vi "Write.Data.vi"(8 "error in (no error)":errorcluster, 10 "Data":u64[](array[numeric]), 11 "FpgaRunner in":refnum<class "FpgaRunner.lvclass">) -> (0 "error out":errorcluster, 3 "FpgaRunner out":refnum<class "FpgaRunner.lvclass">)   [LabVIEW 2020, in "FpgaRunner.lvclass"]
uses:
  FpgaRunner.lvclass
  FpgaRunner.lvclass/FpgaRunner.ctl
  <vilib>/Utility/error.llb/Error Cluster From Error Code.vi
  <vilib>/rvi/errors/niLvFpgaAdjustHostInterfaceError.vi
  <vilib>/rvi/interface/nirviMethod/nirviMethod.xnode
  <vilib>/FPGAPlugInAG/Dynamic/niLvFpga_WriteFifo_Dynamic.vi
  <vilib>/rvi/errors/niLvFpgaMergeErrorWithErrorCode.vi
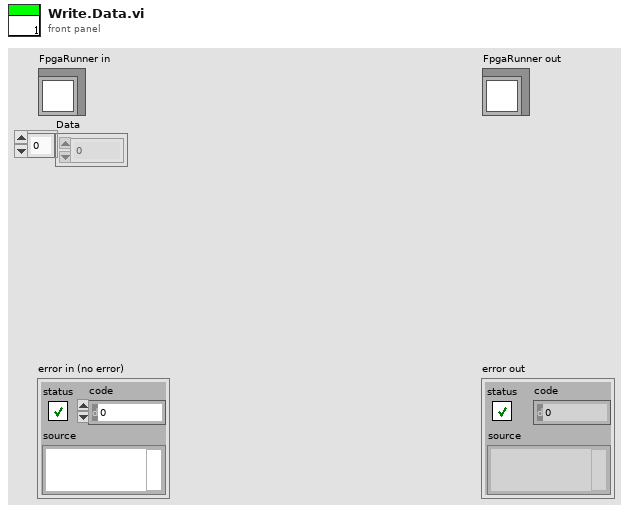
[diagram p1: front panel]
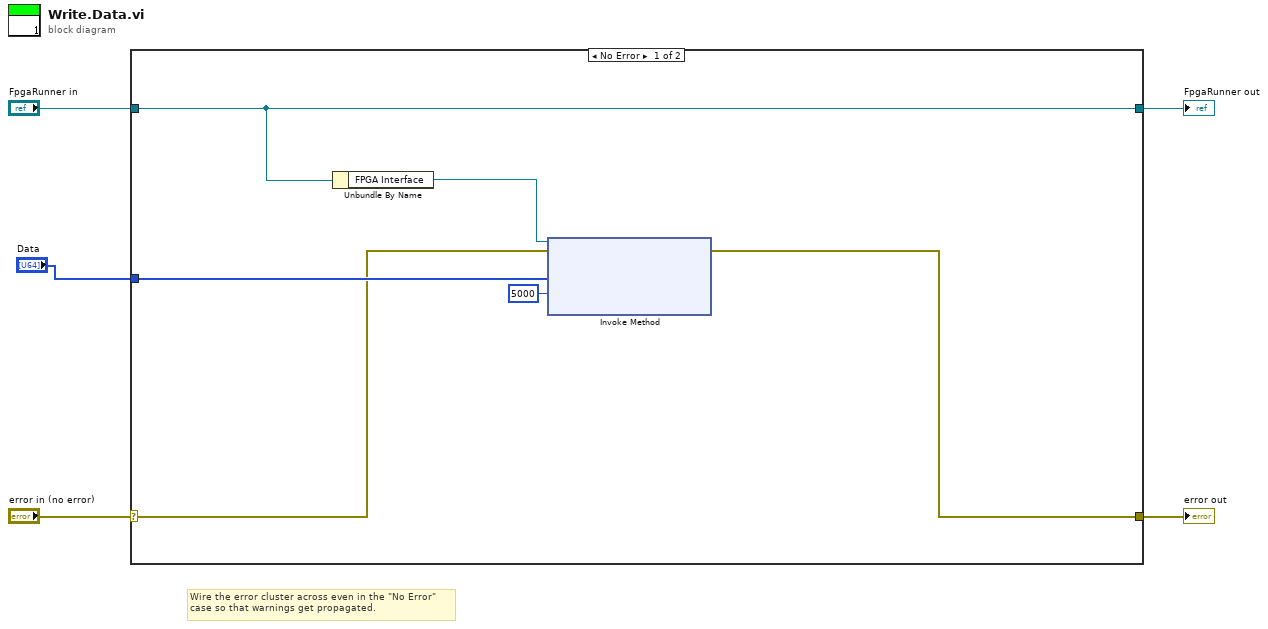
[diagram p0: block diagram]
diagram:
  # "Wire the error cluster across even in the \"No Error\"\ncase so that warnings get propagated."
  n1 = case shown="No Error" "error in (no error)" {
    selector: "error in (no error)" -> [w6 w13]
    tunnel: [w7 w13] -> w4
    tunnel: [w9 w12] -> w2
    tunnel: "FpgaRunner in" -> [w9 w12]
    tunnel: "Data" -> [w10 _]
    frame No Error {
      n2 = Unbundle By Name(w9) -> ("FPGA Interface"=w8:refnum<k20>)
      n3 = xnode "Invoke Method"("FPGA VI Reference In"=w8, "error in"=w6, "Data"=w10, "Timeout (ms)"=5000) -> ("error out"=w7:errorcluster)  [unwired: 2 out]
    }
    frame Error {
    }
  }
  "error out" <- w4
  "FpgaRunner out" <- w2
